vi "Agilent SNA Fetch Data.vi"(4 "Trace":i8=1 min=1 max=99 step=1, 6 "Channel":i8=1 min=1 max=99 step=1, 7 "Agilent SNA & SWP":T2, 8 "error in (no error)":errorcluster, 9 "Formatted Data?":bool, 10 "Data to Read (Data)":enum16{"Data", "Memory"}(ring), 11 "VISA Resource Names":T3) -> (0 "error out":errorcluster, 1 "Display Format":T1, 2 "Data (real+imag)":cdb[](array[numeric]), 3 "dup VISA Resource Names":T3)   [LabVIEW 2011]
doc: "It is recommended that you hold off triggers before running this VI as the HP8753 tends to \"hang\" if data is read while measurements are being taken.\n\n This VI is used to collect and display data generated by the HP8753 Network Analyzer. The VI can display error-corrected data, error-corrected trace memory, fully formatted data and memory traces. For further information on these types of data see Processsing Chain figure in the HPIB programming note. When the data type is a formatted data, the instruments screen will change to reflect what is being displayed, eg. selecting \"formatted memory\" changes the display to \"MEMORY\".\n\n The data values shown depend upon the data type and the measurement format. If the data type is \"error-corrected data\" or \"error-corrected trace memory\" and/or the measurement format is \"Smith chart\" or \"polar\", the data values are real,imaginary pairs. Otherwise the data values are stimulus,response pairs. These pairs correspond to what is shown in the graphical display.\n\n Data can also be saved to a file with this VI. When saving a file, the stimulus is always shown. The real,imaginary components or the response value are also shown depending upon the data type and the measurement format. \n\n No units are shown on the VI front panel or in the data file. All units are basic units of Hz, dB, seconds, ohms, etc. The \"saved data comments\" control should be used for any special information such as the measurement format, averaging and smoothing information, etc.\n\n Whether or not data is saved and whether the output is in real,imaginary pairs or stimulus,response parirs affects the speed of this VI. When data is saved to a file and/or when data is in stimulus,response pairs, requires the reading of the stimulus values which slows the VI down. The fastest reads are done when the data type is \"error-corrected data\" or \"error-corrected trace memory\" and/or the measurement format is \"Smith chart\" or \"polar\" and data is not being saved to a file.\n\n This VI sets the format, ie. linear or logarithmic, depending upon the sweep type. \n\nFYI - Originally this VI was written without considering the stimulus values. In most case this would be fine for display purposes as the point number could be used for the X value as most sweeps are evenly spaced. This is not the case with frequency list sweeps which can have big gaps in the sweep. For this reason the stimulus value is read (at least in the cases explained above) to make the LabVIEW display match what is display on the instrument's display."
uses:
  TypeDefs/Agilent SNA VISA.ctl
  TypeDefs/Agilent SNA Instrument Info.ctl
  tests/S Parameter/TypeDefs/SP Measurement Format.ctl
  SNA Measurement Format.ctl
panel:
  out "#data points":i16
  out "bytes to read\n(divide this number\nby 2 bytes per point\nto get # points for\na sanity check)":i16
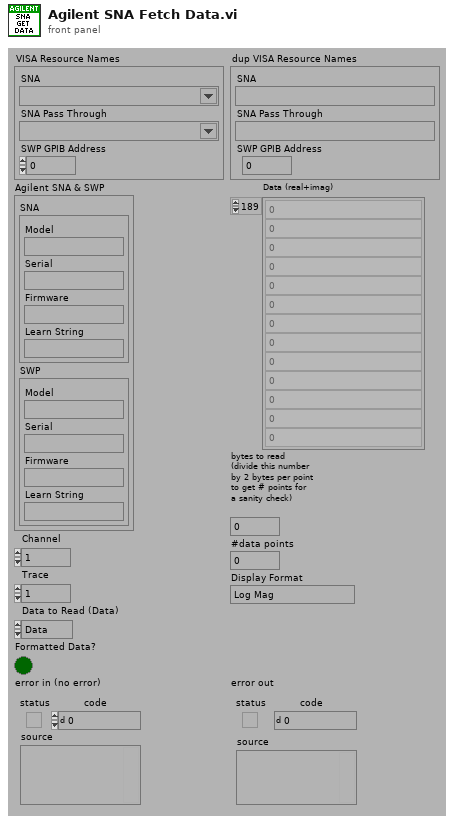
[diagram p1: front panel]
types:
  T1 = typedef "SP Measurement Format.ctl" = enum32{"Log Mag", "Phase", "Delay", "Smith (R+jX)", "Polar (Re/Im)", "Linear Mag", "SWR", "Real", "Imaginary", "Smith (Lin/Phase)", "Smith (Log/Phase)", "Smith (Real/Imag)", "Smith (G+jB)", "Polar (Lin/Phase)", "Polar (Log/Phase)", "Expanded Phase", "Positive Phase", "Inverted Smith", "Unwrapped Phase", "Power Out", "Power In", "Linear Mag/Phase", "Log Mag/Phase", "Real/Imaginary"}
  T2 = typedef "Agilent SNA Instrument Info.ctl" = cluster{"SNA":cluster{"Model":string, "Serial":string, "Firmware":string, "Learn String":string}, "SWP":cluster{"Model":string, "Serial":string, "Firmware":string, "Learn String":string}}
  T3 = typedef "Agilent SNA VISA.ctl" = cluster{"SNA":refnum<visa-resource-name>, "SNA Pass Through":refnum<visa-resource-name>, "SWP GPIB Address":i32}
  T4 = typedef "SNA Measurement Format.ctl" = enum32{"Log Mag", "Normalized Log Mag", "SWR", "Linear Mag", "Power Out"}
  T5 = typedef "Agilent SNA Model.ctl" = enum16{"Not Supported", "8757X"}
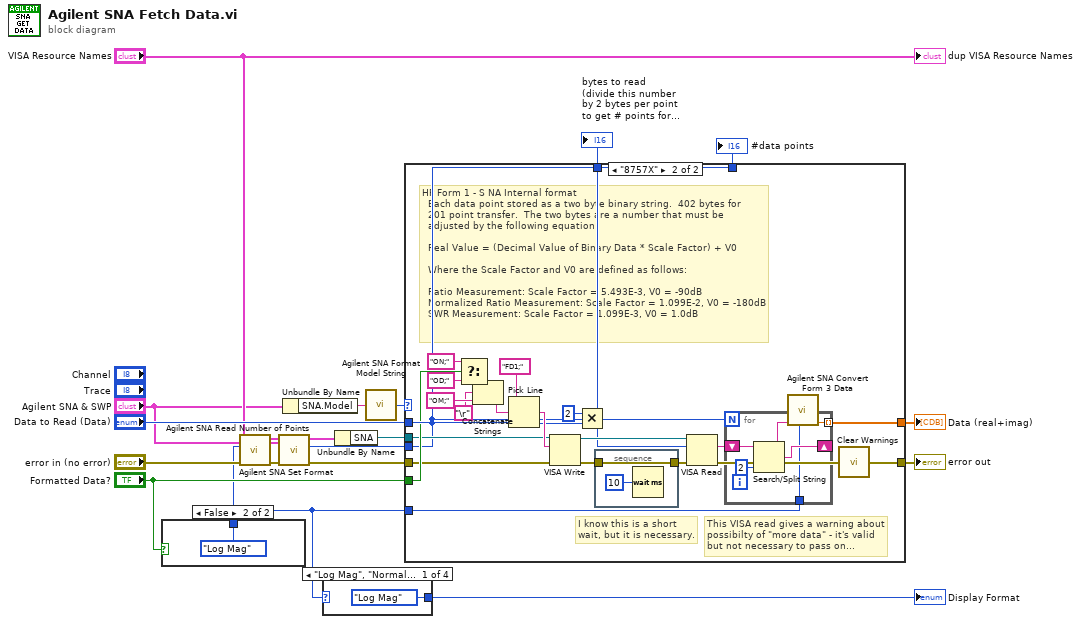
[diagram p0: block diagram]
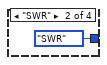
[diagram p2: hidden frame]
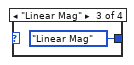
[diagram p3: hidden frame]
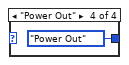
[diagram p4: hidden frame]
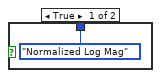
[diagram p5: hidden frame]
diagram:
  n1 = case shown="False" "Formatted Data?" {
    tunnel: [SNA_Measurement_Format."Normalized Log Mag" ("Display Format") SNA_Measurement_Format."Log Mag" ("Display Format")] -> w2
    frame True {
    }
    frame False {
    }
  }
  n2 = call "Agilent SNA Set Format.vi"("Agilent SNA & SWP"="Agilent SNA & SWP", "error in (no error)"="error in (no error)", "Display Format"=w2, "VISA Resource Names"="VISA Resource Names") -> ("error out"=w9:errorcluster, "dup VISA Resource Names"=w6:T3)  [unwired: 1 in, 5 out]
  n3 = call "Agilent SNA Read Number of Points.vi"("Agilent SNA & SWP"="Agilent SNA & SWP", "error in (no error)"=w9, "VISA Resource Names"=w6) -> ("error out"=w8:errorcluster, "Number Points"=w4:i32, "dup VISA Resource Names"=w7:T3)  [unwired: 1 in, 5 out]
  n4 = Unbundle By Name("Agilent SNA & SWP") -> ("SNA.Model"=w12:string)
  n5 = case shown="\"Log Mag\", \"Normalized Log Mag\", Default" w2 {
    tunnel: [SP_Measurement_Format."Log Mag" ("Display Format") SP_Measurement_Format."SWR" ("Display Format") SP_Measurement_Format."Linear Mag" ("Display Format") SP_Measurement_Format."Power Out" ("Display Format")] -> w1
    frame "Log Mag", "Normalized Log Mag", Default {
    }
    frame "SWR" {
    }
    frame "Linear Mag" {
    }
    frame "Power Out" {
    }
  }
  "Display Format" <- w1
  n6 = Unbundle By Name(w7) -> ("SNA"=w11:refnum<visa-resource-name>)
  n7 = call "Agilent SNA Format Model String.vi"("Model String"=w12) -> ("Model"=w18:T5)
  n8 = case shown="\"8757X\"" w18 {
    tunnel: w11 -> [_ w35]
    tunnel: w8 -> [w26 w29]
    tunnel: [w26 w30] -> w13
    tunnel: [_ w39] -> w19
    tunnel: "Data to Read (Data)" -> [_ w48]
    tunnel: w2 -> [_ w37]
    tunnel: "Formatted Data?" -> [_ w38]
    tunnel: [_ w33] -> w15
    tunnel: [_ w31] -> w14
    tunnel: w4 -> [_ w33]
    frame "Not Supported" {
    }
    frame "8757X" {
      # "I know this is a short\nwait, but it is necessary."
      # "This VISA read gives a warning about\npossibilty of \"more data\" - it's valid\nbut not necessary to pass on..."
      # "HP Form 1 - S NA Internal format\n  Each data point stored as a two byte binary string.  402 bytes for\n  201 point transfer.  The two bytes are a number that must be\n  adjusted by the following equation:\n\n  Real Value = (Decimal Value of Binary Data * Scale Factor) + V0\n\n  Where the Scale Factor and V0 are defined as follows:\n\n  Ratio Measurement: Scale Factor = 5.493E-3, V0 = -90dB\n  Normalized Ratio Measurement: Scale Factor = 1.099E-2, V0 = -180dB\n  SWR Measurement: Scale Factor = 1.099E-3, V0 = 1.0dB"
      n9 = Select(t="ON;", s=w38, f="OD;") -> (s? t:f=w41:string)
      n10 = Concatenate Strings(w41, "\r", "OM;") -> (w45:string)
      n11 = Pick Line(string ("")="FD1;", multi-line string=w45, line index=w48) -> (output string=w47:string)
      n12 = VISA Write(VISA resource name=w35, write buffer=w47, error in (no error)=w29) -> (VISA resource name out=w34:refnum<visa-resource-name>, error out=w28:errorcluster)  [unwired: 1 out]
      n13 = Multiply(x=2, y=w33) -> (x*y=w31:i32)
      n14 = stacked-sequence {
        tunnel: w28 -> [w50]
        tunnel: [w50] -> w27
        frame #0 {
          n15 = Wait (ms)(milliseconds to wait=u32 10) -> ()  [unwired: 1 out]
        }
      }
      n16 = VISA Read(VISA resource name=w34, byte count=w31, error in (no error)=w27) -> (read buffer=w49:string, error out=w36:errorcluster)  [unwired: 2 out]
      n17 = for {
        N: w33 -> [_]
        shift-right: [w56] -> _
        shift-left: w49 -> [w57]
        tunnel: [w53] -> w39 mode=indexing
        tunnel: w37 -> [w52]
        n18 = Search/Split String(string=w57, offset (0)=2) -> (substring before match=w54:string, match + rest of string=w56:string)  [unwired: 2 out]
        n19 = call "Agilent SNA Convert Form 3 Data.vi"("Measurement Format (Log Mag)"=w52, "Raw Data Point"=w54) -> ("Number"=w53:cdb)  [unwired: 9 out]
      }
      n20 = call "Clear Warnings.vi"("error in (no error)"=w36) -> ("error out"=w30:errorcluster)
    }
  }
  "error out" <- w13
  "Data (real+imag)" <- w19
  "bytes to read\n(divide this number\nby 2 bytes per point\nto get # points for\na sanity check)" <- w14
  "#data points" <- w15
  "dup VISA Resource Names" <- "VISA Resource Names"
